vi "unpack.vi"(6 "超时时间":u32=3000, 7 "串口号输入":refnum<visa-resource-name>) -> (2 "告警信息":string, 3 "应答":string)   [LabVIEW 2014]
panel:
  out "读取缓冲区":string
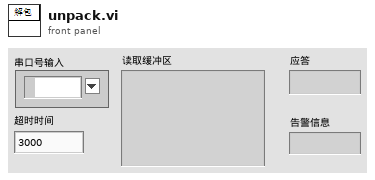
[diagram p1: front panel]
types:
  T1 = cluster{"有功常数":i32, "无功常数":i32, "校验圈数":i32, "校验类型":i32, "S值计算次数":i32, "S值计算方法":i32}
  T2 = cluster{"有功功率":sgl, "有功电能":sgl, "有功脉冲":u64, "标准偏差值":sgl[], "电能误差":sgl[], "脉冲输入功率":sgl[], "脉冲电能累计":sgl[], "输入脉冲数":sgl[]}
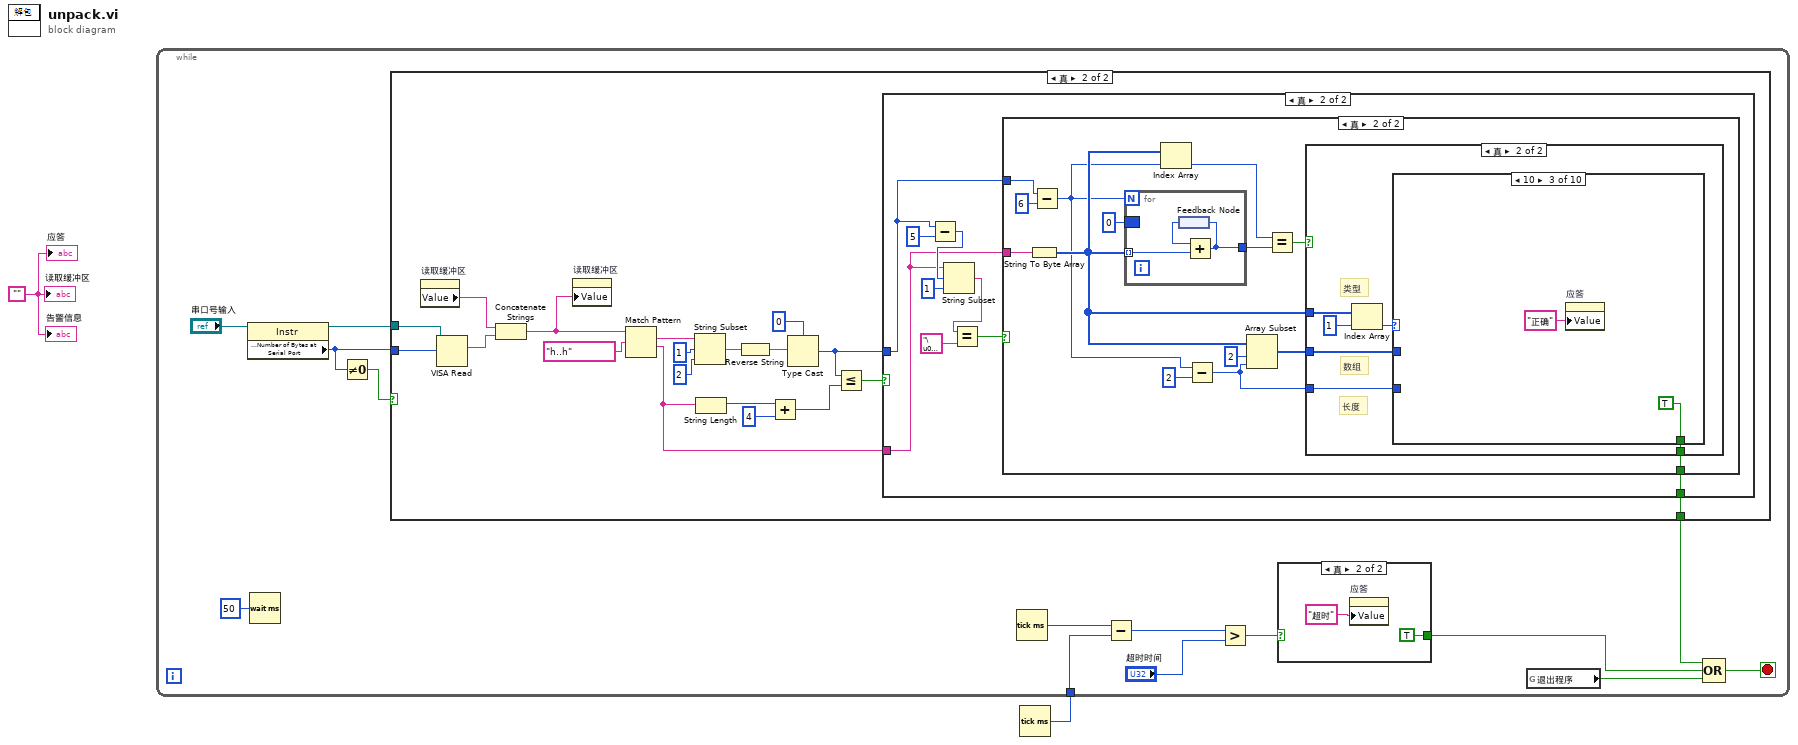
[diagram p0: block diagram]
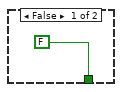
[diagram p3: hidden frame]
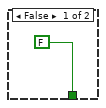
[diagram p4: hidden frame]
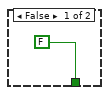
[diagram p5: hidden frame]
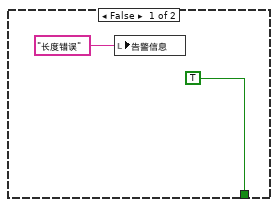
[diagram p6: hidden frame]
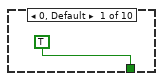
[diagram p7: hidden frame]
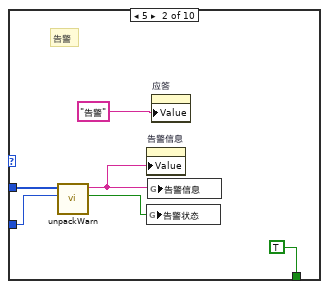
[diagram p8: hidden frame]
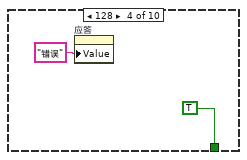
[diagram p9: hidden frame]
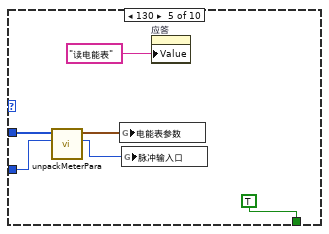
[diagram p10: hidden frame]
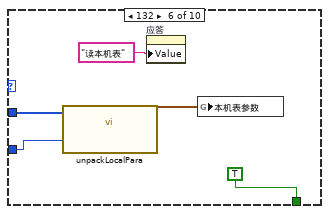
[diagram p11: hidden frame]
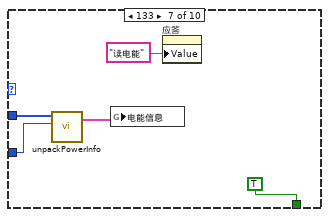
[diagram p12: hidden frame]
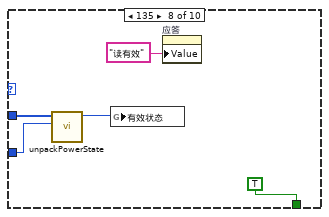
[diagram p13: hidden frame]
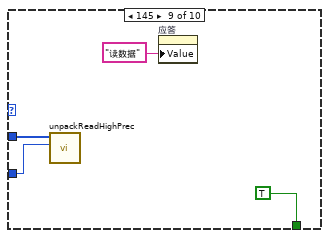
[diagram p14: hidden frame]
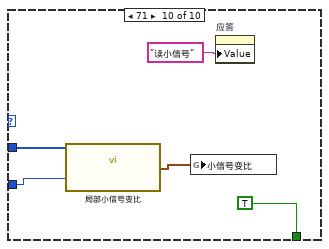
[diagram p15: hidden frame]
diagram:
  w1 = "" ("读取缓冲区")
  n1 = Tick Count (ms)() -> (millisecond timer value=w2:u32)
  n2 = while {
    tunnel: w2 -> [w7]
    stop <- w3 stop-if-true
    n3 = property class="Instr"(reference="串口号输入") -> (reference out=w14:refnum<visa-resource-name>, "Serial Settings:Number of Bytes at Serial Port"=w9:u32)  [unwired: 1 in, 1 out]
    n4 = Wait (ms)(milliseconds to wait=u32 50 ("等待时间（毫秒）")) -> ()  [unwired: 1 out]
    n5 = Not Equal To 0?(x=w9) -> (x != 0?=w15:bool)
    n6 = case shown="真" w15 {
      tunnel: w14 -> [_ w39]
      tunnel: [FALSE w28] -> w6
      tunnel: w9 -> [_ w27]
      frame False {
      }
      frame True {
        n7 = property on="读取缓冲区" class="Str"() -> ("Value"=w38:string)  [unwired: 2 in, 2 out]
        n8 = VISA Read(VISA resource name=w39, byte count=w27) -> (read buffer=w26:string)  [unwired: 1 in, 3 out]
        n9 = Concatenate Strings(w38, w26) -> (w25:string)
        n10 = property on="读取缓冲区" class="Str"("Value"=w25) -> ()  [unwired: 2 in, 2 out]
        n11 = Match Pattern(string=w25, regular expression="h..h" ("正则表达式")) -> (match substring=w24:string, after substring=w23:string)  [unwired: 1 in, 2 out]
        n12 = String Subset(string=w24, offset (0)=1 ("偏移量(0)"), length (rest)=2 ("长度（剩余）")) -> (substring=w22:string)
        n13 = String Length(string=w23) -> (length=w33:i32)
        n14 = Reverse String(1:w22) -> (0:w21:string)
        n15 = Add(x=w33, y=4) -> (x+y=w31:i32)
        n16 = Type Cast(type=u16 0, x=w21) -> (*(type *) &x=w30:u16)
        n17 = Less Or Equal?(x=w30, y=w31) -> (x <= y?=w29:bool)
        n18 = case shown="真" w29 {
          tunnel: w23 -> [_ w42]
          tunnel: w30 -> [_ w43]
          tunnel: [FALSE w41] -> w28
          frame False {
          }
          frame True {
            n19 = Subtract(x=w43, y=5) -> (x-y=w46:i32)
            n20 = String Subset(string=w42, offset (0)=w46, length (rest)=1 ("长度（剩余）")) -> (substring=w48:string)
            n21 = Equal?(x=w48, y="\u0016") -> (x = y?=w44:bool)
            n22 = case shown="真" w44 {
              tunnel: w43 -> [_ w55]
              tunnel: w42 -> [_ w63]
              tunnel: [FALSE w58] -> w41
              frame False {
              }
              frame True {
                n23 = String To Byte Array(string=w63) -> (unsigned byte array=w57:u8[])
                n24 = Subtract(x=w55, y=6) -> (x-y=w52:i32)
                n25 = for {
                  N: w52 -> [_]
                  tunnel: w57 -> [w116] mode=indexing
                  border: u8 0 -> [_]
                  tunnel: [w114] -> w60
                  n26 = feedback #1() -> (w115:u8)
                  n27 = Add(x=w115, y=w116) -> (x+y=w114:u8)
                  n28 = feedback-in #1(w114) -> ()
                }
                n29 = Index Array(array=w57, index=w52) -> (element=w61:u8)
                n30 = Subtract(x=w52, y=2) -> (x-y=w51:i32)
                n31 = Array Subset(array=w57, index=2 ("索引"), length=w51) -> (w53:u8[])
                n32 = Equal?(x=w61, y=w60) -> (x = y?=w59:bool)
                n33 = case shown="真" w59 {
                  tunnel: w57 -> [_ w70]
                  tunnel: [TRUE w69] -> w58
                  tunnel: w53 -> [_ w68]
                  tunnel: w51 -> [_ w67]
                  frame False {
                    n34 = local write "告警信息"("长度错误") -> ()
                  }
                  frame True {
                    # "类型"
                    # "数组"
                    # "长度"
                    n35 = Index Array(array=w70, index=1 ("索引")) -> (element=w71:u8)
                    n36 = case shown="10" w71 {
                      tunnel: [TRUE TRUE TRUE TRUE TRUE TRUE TRUE TRUE TRUE TRUE] -> w69
                      tunnel: w68 -> [_ w78 _ _ w89 w94 w99 w104 w107 w113]
                      tunnel: w67 -> [_ w77 _ _ w88 w93 w98 w103 w106 w112]
                      frame 0, Default {
                      }
                      frame 5 {
                        # "告警"
                        n37 = call "unpackWarn.vi"("长度"=w77, "数据"=w78) -> ("告警状态"=w75:bool, "告警信息"=w74:string)  [unwired: 4 in]
                        n38 = property on="告警信息" class="Str"("Value"=w74) -> ()  [unwired: 2 in, 2 out]
                        n39 = global write "系统全局.vi" "告警状态"(w75) -> ()
                        n40 = global write "系统全局.vi" "告警信息"(w74) -> ()
                        n41 = property on="应答" class="Str"("Value"="告警" ("字符串")) -> ()  [unwired: 2 in, 2 out]
                      }
                      frame 16 {
                        n42 = property on="应答" class="Str"("Value"="正确" ("字符串")) -> ()  [unwired: 2 in, 2 out]
                      }
                      frame 128 {
                        n43 = property on="应答" class="Str"("Value"="错误" ("字符串")) -> ()  [unwired: 2 in, 2 out]
                      }
                      frame 130 {
                        n44 = call "unpackMeterPara.vi"("长度"=w88, "数据"=w89) -> ("输入通道"=w86:u8, "电能表参数"=w87:T1)  [unwired: 4 in]
                        n45 = global write "程序全局.vi" "电能表参数"(w87) -> ()
                        n46 = global write "程序全局.vi" "脉冲输入口"(w86) -> ()
                        n47 = property on="应答" class="Str"("Value"="读电能表" ("字符串")) -> ()  [unwired: 2 in, 2 out]
                      }
                      frame 132 {
                        n48 = call "unpackLocalPara.vi"("长度"=w93, "数据"=w94) -> ("本机表参数"=w91:cluster{"有功常数":i32, "无功常数":i32, "输出类型":i32})  [unwired: 4 in, 1 out]
                        n49 = property on="应答" class="Str"("Value"="读本机表" ("字符串")) -> ()  [unwired: 2 in, 2 out]
                        n50 = global write "程序全局.vi" "本机表参数"(w91) -> ()
                      }
                      frame 133 {
                        n51 = call "unpackPowerInfo.vi"("长度"=w98, "数据"=w99) -> ("电能信息"=w95:T2)  [unwired: 3 in]
                        n52 = global write "程序全局.vi" "电能信息"(w95) -> ()
                        n53 = property on="应答" class="Str"("Value"="读电能" ("字符串")) -> ()  [unwired: 2 in, 2 out]
                      }
                      frame 135 {
                        n54 = call "unpackPowerState.vi"("长度"=w103, "数据"=w104) -> ("有效状态"=w100:u8)  [unwired: 4 in, 1 out]
                        n55 = global write "程序全局.vi" "有效状态"(w100) -> ()
                        n56 = property on="应答" class="Str"("Value"="读有效" ("字符串")) -> ()  [unwired: 2 in, 2 out]
                      }
                      frame 145 {
                        n57 = call "unpackReadHighPrec.vi"("长度"=w106, "数据"=w107) -> ()  [unwired: 3 in, 1 out]
                        n58 = property on="应答" class="Str"("Value"="读数据" ("字符串")) -> ()  [unwired: 2 in, 2 out]
                      }
                      frame 71 {
                        n59 = call "局部小信号变比.vi"("长度"=w112, "数据"=w113) -> ("小信号变比"=w109:cluster{"UB":sgl, "IB":sgl, "UC":sgl})  [unwired: 3 in]
                        n60 = global write "程序全局.vi" "小信号变比"(w109) -> ()
                        n61 = property on="应答" class="Str"("Value"="读小信号" ("字符串")) -> ()  [unwired: 2 in, 2 out]
                      }
                    }
                  }
                }
              }
            }
          }
        }
      }
    }
    n62 = Tick Count (ms)() -> (millisecond timer value=w13:u32)
    n63 = Subtract(x=w13, y=w7) -> (x-y=w11:u32)
    n64 = Greater?(x=w11, y="超时时间") -> (0:w10:bool)
    n65 = case shown="真" w10 {
      selector: w10 -> [w17 _]
      tunnel: [w17 TRUE] -> w5
      frame False {
      }
      frame True {
        n66 = property on="应答" class="Str"("Value"="超时" ("字符串")) -> ()  [unwired: 2 in, 2 out]
      }
    }
    n67 = global read "系统全局.vi" "退出程序"() -> (w4:bool)
    n68 = Compound Arithmetic op=OR(w6, w5, w4) -> (w3:bool)
  }
  "读取缓冲区" <- w1
  "应答" <- w1
  "告警信息" <- w1
